vi "Get base paths.vi"(8 "error in (no error)":errorcluster, 11 "DAQOrcaFlash in":refnum<class "DAQOrcaFlash.lvclass">) -> (0 "error out":errorcluster, 1 "final conversion folder":path, 2 "filepath":path, 3 "DAQOrcaFlash out":refnum<class "DAQOrcaFlash.lvclass">)   [LabVIEW 2012, in "DAQOrcaFlash.lvclass"]
uses:
  DAQOrcaFlash.lvclass
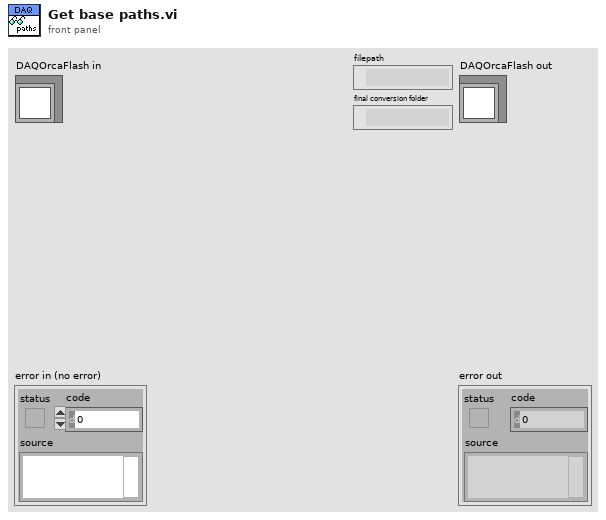
[diagram p1: front panel]
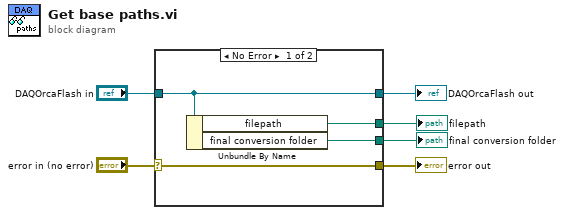
[diagram p0: block diagram]
diagram:
  n1 = case shown="No Error" "error in (no error)" {
    selector: "error in (no error)" -> [w10 w12]
    tunnel: [w10 w12] -> w5
    tunnel: [w9 w11] -> w3
    tunnel: "DAQOrcaFlash in" -> [w9 w11]
    tunnel: [w8 _] -> w2
    tunnel: [w7 _] -> w1
    frame No Error {
      n2 = Unbundle By Name(w9) -> ("filepath"=w8:path, "final conversion folder"=w7:path)
    }
    frame Error {
    }
  }
  "error out" <- w5
  "DAQOrcaFlash out" <- w3
  "filepath" <- w2
  "final conversion folder" <- w1
